vi "Tree Copy Single Item.vi"(6 "Parent Tag":string, 8 "error in":errorcluster, 9 "Target Tree Ref In":refnum<vi>, 10 "Target Item":string, 11 "Source Tree Ref In":refnum<vi>) -> (0 "error out":errorcluster, 1 "Target Tree Ref Out":refnum<vi>, 3 "Source Tree Ref Out":refnum<vi>)   [LabVIEW 2024]
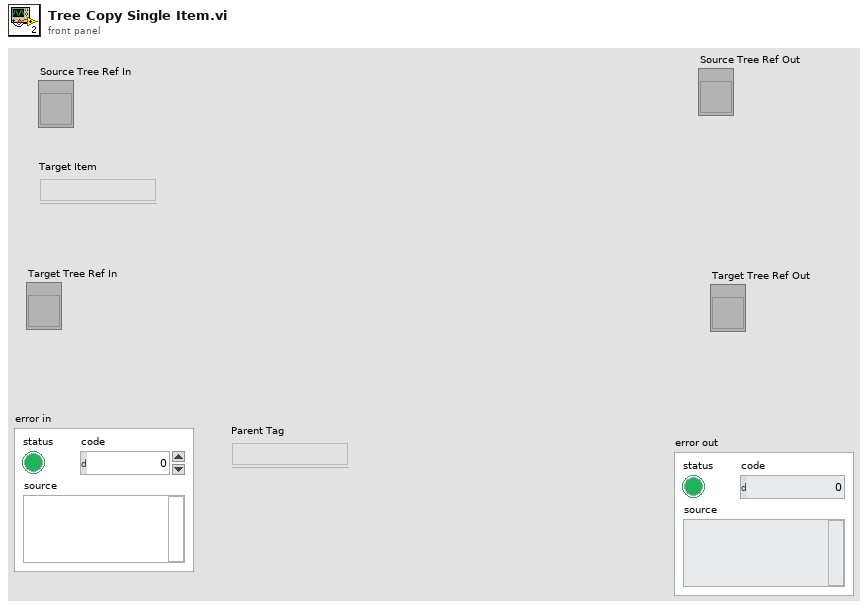
[diagram p1: front panel]
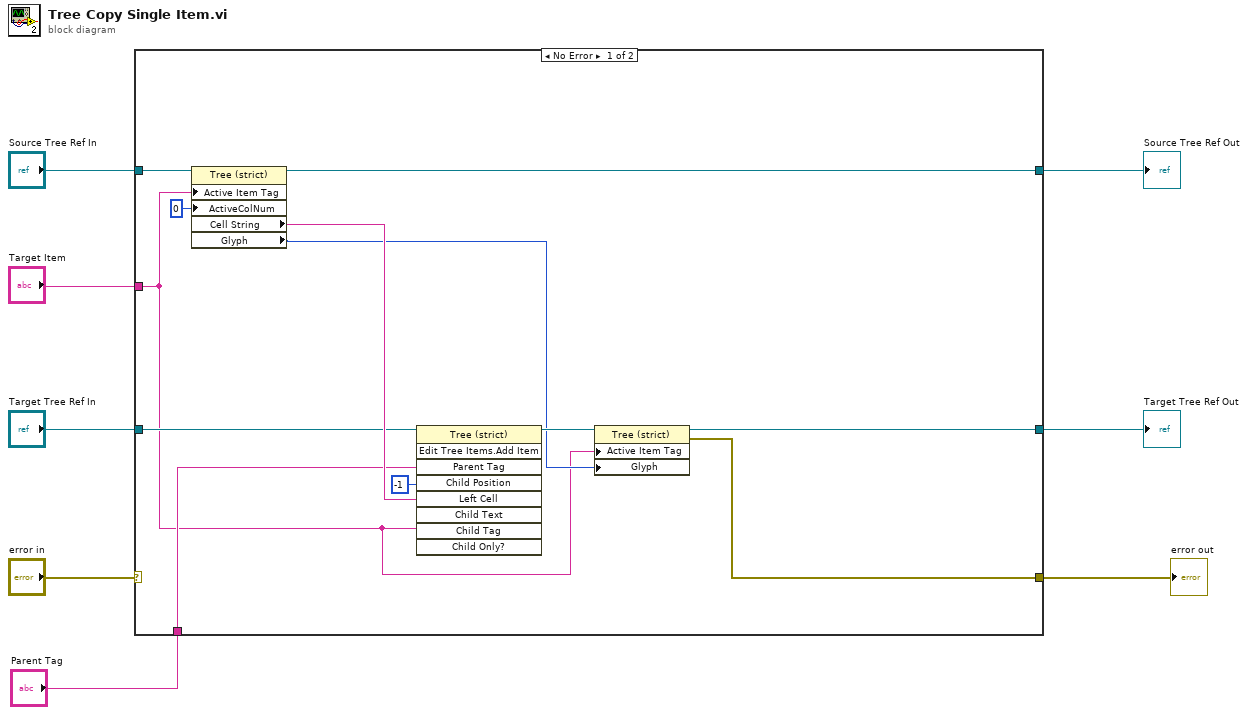
[diagram p0: block diagram]
diagram:
  n1 = case shown="No Error" "error in" {
    selector: "error in" -> [_ w23]
    tunnel: [w12 w23] -> w7
    tunnel: "Target Tree Ref In" -> [w15 w21]
    tunnel: "Target Item" -> [w10 _]
    tunnel: "Source Tree Ref In" -> [w20 w22]
    tunnel: "Parent Tag" -> [w11 _]
    tunnel: [w14 w22] -> w2
    tunnel: [w13 w21] -> w1
    frame No Error {
      n2 = property class="Tree (strict)"(reference=w20, "Active Item Tag"=w10, "ActiveColNum"=0 ("Active Cell:Active Column Number")) -> (reference out=w14:refnum<vi>, "Cell String"=w18:string, "Glyph"=w16:i32)  [unwired: 1 in, 1 out]
      n3 = invoke class="Tree (strict)" method="Edit Tree Items.Add Item"(reference=w15, "Parent Tag"=w11, "Child Position"=-1, "Left Cell"=w18, "Child Tag"=w10) -> (reference out=w17:refnum<vi>)  [unwired: 4 in, 8 out]
      n4 = property class="Tree (strict)"(reference=w17, "Active Item Tag"=w10, "Glyph"=w16) -> (reference out=w13:refnum<vi>, error out=w12:errorcluster)  [unwired: 1 in]
    }
    frame Error {
    }
  }
  "Source Tree Ref Out" <- w2
  "Target Tree Ref Out" <- w1
  "error out" <- w7
